vi "F Dwf Analog In Channel Range Set.vi"(8 "error in (no error)":errorcluster, 9 "voltsRange":dbl, 10 "idxChannel":i32, 11 "hdwf":i32) -> (0 "error out":errorcluster, 3 "function return":i32)   [LabVIEW 2021, in "Olasdwf.lvlib"]
doc: "DWFAPI int FDwfAnalogInChannelRangeSet(HDWF hdwf, int idxChannel, double voltsRange);"
uses:
  Olasdwf.lvlib
  Windows/System32/dwf.dll
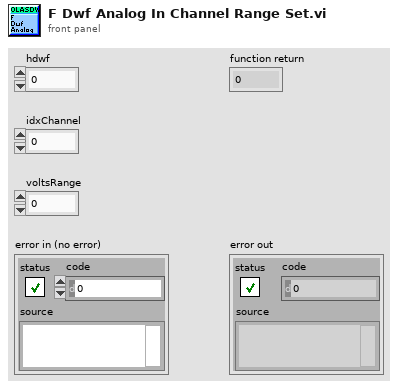
[diagram p1: front panel]
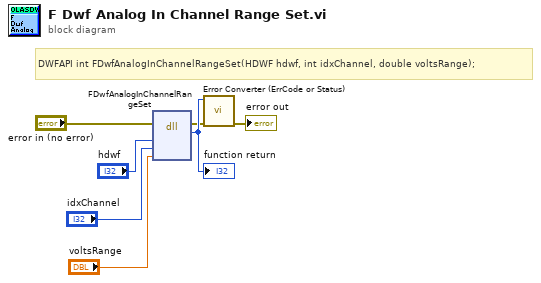
[diagram p0: block diagram]
diagram:
  # "DWFAPI int FDwfAnalogInChannelRangeSet(HDWF hdwf, int idxChannel, double voltsRange);"
  n1 = dll-call lib="/Windows/System32/dwf.*" fn="FDwfAnalogInChannelRangeSet"(error in="error in (no error)", "hdwf"="hdwf", "idxChannel"="idxChannel", "voltsRange"="voltsRange") -> (error out=w2:errorcluster, w7:i32)  [unwired: 5 in, 1 out]
  "function return" <- w7
  n2 = call "Error Converter (ErrCode or Status).vi"("error in (no error)"=w2, "error code"=w7) -> ("error out"=→"error out":errorcluster)  [unwired: 9 in]
